vi "Subvi_PolyItemTemp.vi"() -> ()   [LabVIEW 2015]
uses:
  C:/Users/jeff.lin.MINAIK/Desktop/Scripting/Control_MessageCluster.ctl
  C:/Users/jeff.lin.MINAIK/Desktop/Scripting/Control_QueueMessage.ctl
  C:/Users/jeff.lin.MINAIK/Desktop/Scripting/Control_Queue.ctl
panel:
  out "element":cluster{"DataName":string, "Variant":variant}
  in  "Queue name":string="UI"
  out "error out":errorcluster
  out "Queue Out":T1
  in  "Queue Control":T2
  in  "error in (no error)":errorcluster
  in  "Queue in":T1
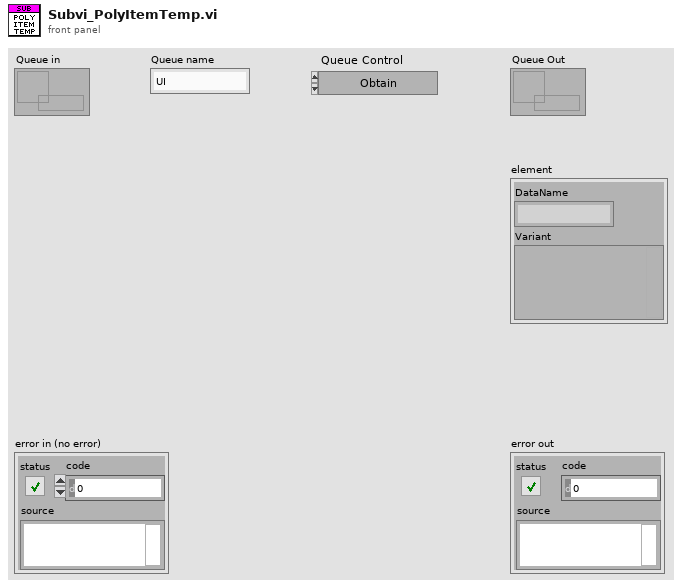
[diagram p1: front panel]
types:
  T1 = typedef "Control_QueueMessage.ctl" = refnum<queue>
  T2 = typedef "Control_Queue.ctl" = enum16{"Obtain", "Enqueue", "Enqueue (End)", "Dequeue", "Flush", "Release"}
  T3 = typedef "Control_MessageCluster.ctl" = cluster{"Message":string, "Message Data":variant}
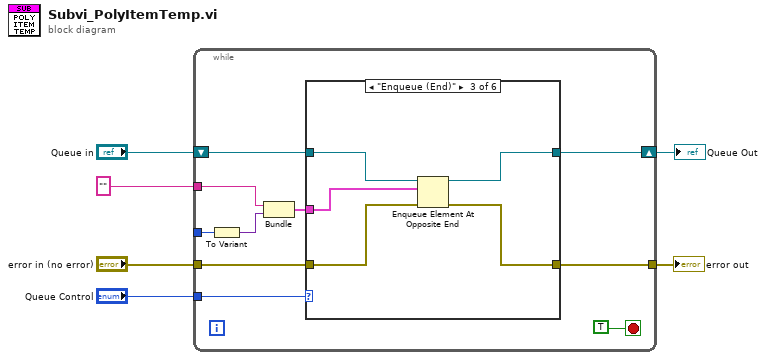
[diagram p0: block diagram]
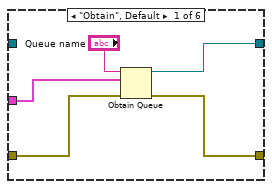
[diagram p2: hidden frame]
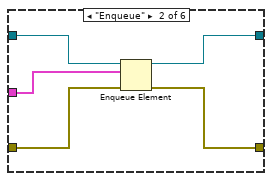
[diagram p3: hidden frame]
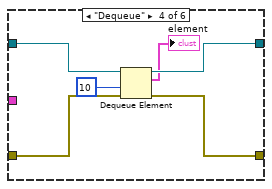
[diagram p4: hidden frame]
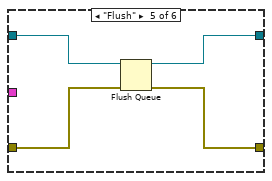
[diagram p5: hidden frame]
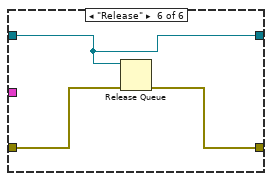
[diagram p6: hidden frame]
diagram:
  n1 = while {
    shift-right: [w7] -> w6
    shift-left: "Queue in" -> [w12]
    tunnel: "Queue Control" -> [w9]
    tunnel: _ -> [w15]
    tunnel: "error in (no error)" -> [w10]
    tunnel: "" -> [w14]
    tunnel: [w8] -> w1
    stop <- TRUE stop-if-true
    n2 = To Variant(anything=w15) -> (Variant=w13:variant)
    n3 = Bundle(w14, "Variant"=w13) -> (w11:cluster{string, "Variant":variant})  [unwired: 1 in]
    n4 = case shown="\"Enqueue (End)\"" w9 {
      tunnel: w10 -> [w21 w23 w28 w35 w38 w43]
      tunnel: [w20 w24 w29 w34 w39 w44] -> w8
      tunnel: [w19 w25 w30 w36 w40 w42] -> w7
      tunnel: w12 -> [_ w26 w31 w37 w41 w42]
      tunnel: w11 -> [w18 w22 w27 _ _ _]
      frame "Obtain", Default {
        n5 = Obtain Queue(name (unnamed)="Queue name", element data type=w18, error in (no error)=w21) -> (queue out=w19:refnum<queue>, error out=w20:errorcluster)  [unwired: 2 in, 1 out]
      }
      frame "Enqueue" {
        n6 = Enqueue Element(queue=w26, element=w22, error in (no error)=w23) -> (queue out=w25:T1, error out=w24:errorcluster)  [unwired: 1 in, 1 out]
      }
      frame "Enqueue (End)" {
        n7 = Enqueue Element At Opposite End(queue=w31, element=w27, error in (no error)=w28) -> (queue out=w30:T1, error out=w29:errorcluster)  [unwired: 1 in, 1 out]
      }
      frame "Dequeue" {
        n8 = Dequeue Element(queue=w37, timeout in ms (-1)=10, error in (no error)=w35) -> (queue out=w36:T1, element=→"element":T3, error out=w34:errorcluster)  [unwired: 1 out]
      }
      frame "Flush" {
        n9 = Flush Queue(queue=w41, error in (no error)=w38) -> (queue out=w40:T1, error out=w39:errorcluster)  [unwired: 1 out]
      }
      frame "Release" {
        n10 = Release Queue(queue=w42, error in (no error)=w43) -> (error out=w44:errorcluster)  [unwired: 1 in, 2 out]
      }
    }
  }
  "Queue Out" <- w6
  "error out" <- w1
